vi "Frame Command Data Command.vi"(11 "DAC channel":u32 caption="DAC CHANNEL") -> (3 "Command_Data array":i16[](array[numeric]))   [LabVIEW 2021]
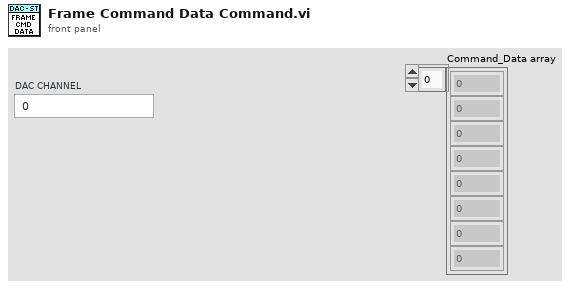
[diagram p1: front panel]
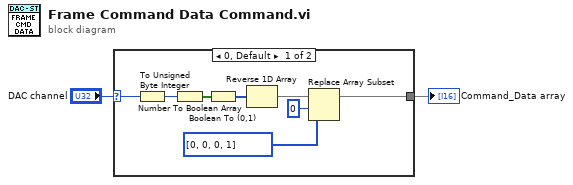
[diagram p0: block diagram]
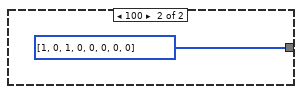
[diagram p2: hidden frame]
diagram:
  n1 = case shown="0, Default" "DAC channel" {
    selector: "DAC channel" -> [w8 _]
    tunnel: [w3 i16[] [1, 0, 1, 0, 0, 0, 0, 0]] -> w1
    frame 0, Default {
      n2 = To Unsigned Byte Integer(number=w8) -> (unsigned 8bit integer=w7:u8)
      n3 = Number To Boolean Array(number=w7) -> (Boolean array=w10:bool[])
      n4 = Boolean To (0,1)(Boolean=w10) -> (0, 1=w9:i16[])
      n5 = Reverse 1D Array(array=w9) -> (reversed array=w6:i16[])
      n6 = Replace Array Subset(array=w6, new element=i16[] [0, 0, 0, 1], index=0) -> (w3:i16[])
    }
    frame 100 {
    }
  }
  "Command_Data array" <- w1
